vi "OAT Demodulation Initial Lp States.vi"(6 "filter":T1={"coefficients"=[], "factor"=1} {"coefficients" format="%.2f"}, 7 "num of orders":i32, 8 "reset? (True)":bool=TRUE, 9 "Lp Image in":dbl[][](array[numeric]), 10 "Lp Real in":dbl[][](array[numeric])) -> (1 "Lp Image":dbl[][](array[numeric]), 2 "Lp Real":dbl[][](array[numeric]))   [LabVIEW 2017, in "SoundVib_Resampling.lvlib"]
uses:
  <vilib>/addons/Sound and Vibration/Order Analysis/Resample Order Tracking/SoundVib_Resampling.lvlib
  <vilib>/addons/_NISVFA/_Shared subVIs/Controls/OAT Decimation Filter.ctl
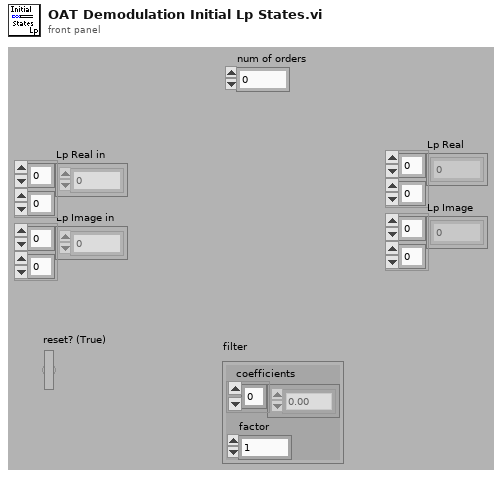
[diagram p1: front panel]
types:
  T1 = typedef "OAT Decimation Filter.ctl" = cluster{"coefficients":dbl[], "factor":i32}
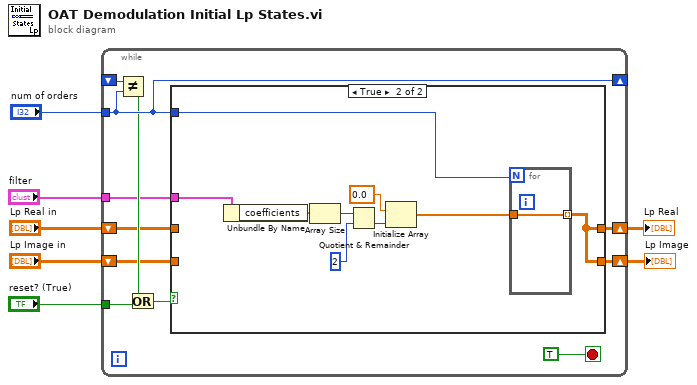
[diagram p0: block diagram]
diagram:
  n1 = while {
    tunnel: "reset? (True)" -> [w15]
    shift-right: [w16] -> _
    shift-left: _ -> [w17]
    tunnel: "num of orders" -> [w16]
    shift-right: [w9] -> w4
    shift-left: "Lp Real in" -> [w12]
    shift-right: [w8] -> w3
    shift-left: "Lp Image in" -> [w11]
    tunnel: "filter" -> [w10]
    stop <- TRUE stop-if-true
    n2 = Not Equal?(x=w17, y=w16) -> (x != y?=w14:bool)
    n3 = Or(x=w14, y=w15) -> (x .or. y?=w13:bool)
    n4 = case shown="True" w13 {
      tunnel: w16 -> [_ w24]
      tunnel: w12 -> [w20 _]
      tunnel: w11 -> [w19 _]
      tunnel: w10 -> [_ w23]
      tunnel: [w20 w22] -> w9
      tunnel: [w19 w22] -> w8
      frame False {
      }
      frame True {
        n5 = Unbundle By Name(w23) -> ("coefficients"=w29:dbl[])
        n6 = Array Size(array=w29) -> (size(s)=w27:i32)
        n7 = Quotient & Remainder(x=w27, y=2 ("Element Data")) -> (floor(x/y)=w26:i32)  [unwired: 1 out]
        n8 = Initialize Array(0.0 ("Element Data"), w26) -> (w21:dbl[])
        n9 = for {
          N: w24 -> [_]
          tunnel: [w30] -> w22 mode=indexing
          tunnel: w21 -> [w30]
        }
      }
    }
  }
  "Lp Real" <- w4
  "Lp Image" <- w3
